vi "HTTP Server Loop.vi"(8 "error in (no error)":errorcluster, 11 "LV Server in":refnum<class "LV Server.lvclass">) -> (0 "error out":errorcluster)   [LabVIEW 2020, in "LV Server.lvclass"]
uses:
  LV Server.lvclass
  lv-http-util/HTTP Utils/Request/Request.lvclass
  lv-http-util/HTTP Utils/Response/Response.lvclass
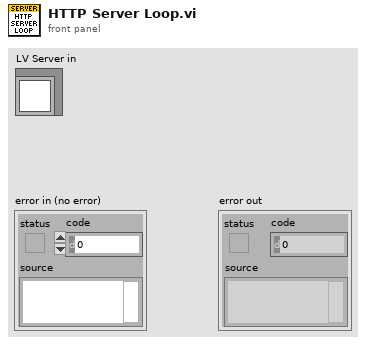
[diagram p1: front panel]
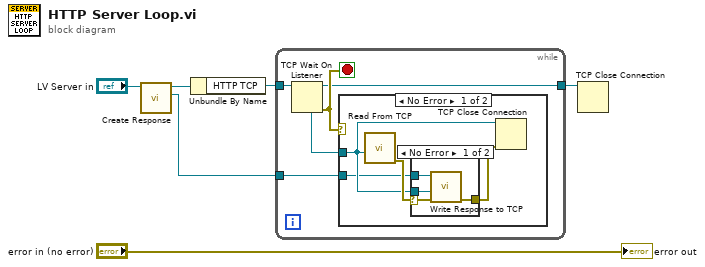
[diagram p0: block diagram]
diagram:
  n1 = call "Create Response.vi"("LV Server in"="LV Server in") -> ("Response out"=w1:refnum<class "Response.lvclass">, "LV Server out"=w2:refnum<class "LV Server.lvclass">)  [unwired: 8 in, 1 out]
  n2 = Unbundle By Name(w2) -> ("HTTP TCP"=w6:refnum<k5>)
  n3 = while {
    tunnel: w6 -> [w11]
    tunnel: w1 -> [w8]
    tunnel: [w7] -> w4
    stop <- w10 stop-if-true
    n4 = TCP Wait On Listener(11:w11) -> (0:w10:errorcluster, 3:w7:refnum<k5>, 4:w9:refnum<k5>)  [unwired: 3 in, 2 out]
    n5 = case shown="No Error" w10 {
      tunnel: w9 -> [w14 _]
      tunnel: w8 -> [w12 _]
      frame No Error {
        n6 = call "Read From TCP.vi"("TCP Connection"=w14) -> ("error out"=w15:errorcluster)  [unwired: 9 in, 1 out]
        n7 = case shown="No Error" w15 {
          selector: w15 -> [w19 w20]
          tunnel: w12 -> [w18 _]
          tunnel: w14 -> [w17 _]
          tunnel: [w16 w20] -> w13
          frame No Error {
            n8 = call "Write Response to TCP.vi"("error in (no error)"=w19, "TCP Connection"=w17, "Response in"=w18) -> ("error out"=w16:errorcluster)  [unwired: 7 in, 1 out]
          }
          frame Error {
          }
        }
        n9 = TCP Close Connection(connection ID=w14, error in (no error)=w13) -> ()  [unwired: 1 in, 2 out]
      }
      frame Error {
      }
    }
  }
  n10 = TCP Close Connection(connection ID=w4) -> ()  [unwired: 2 in, 2 out]
  "error out" <- "error in (no error)"
